vi "single_waveform_array_to_xy_array.vi"(1 "waveform in":waveform(dbl)) -> (0 "XY out":cluster{dbl[], "Y":dbl[]}(graph))   [LabVIEW 2020]
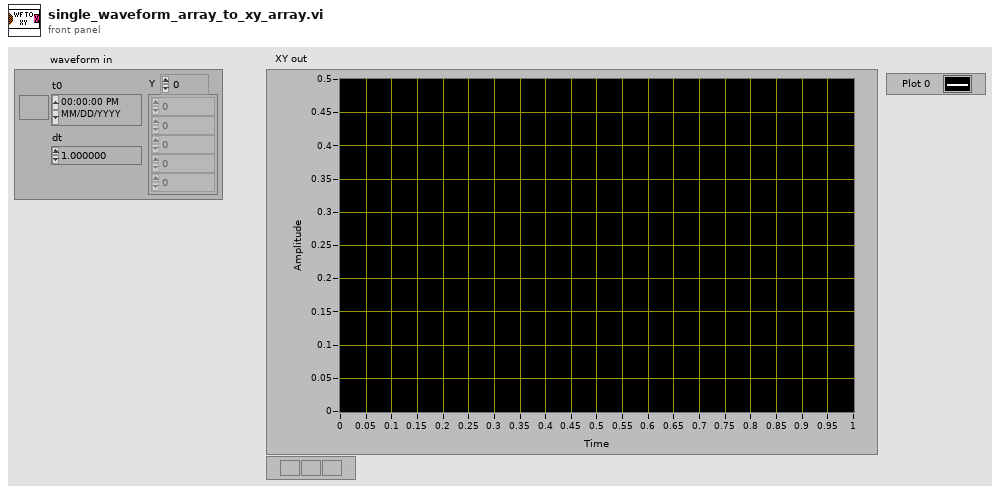
[diagram p1: front panel]
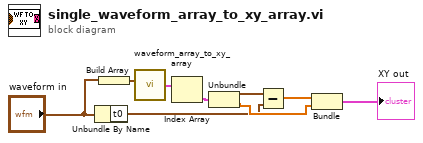
[diagram p0: block diagram]
diagram:
  n1 = Unbundle By Name("waveform in") -> ("t0"=w5:timestamp)
  n2 = Build Array("waveform in") -> (w1:waveform(dbl)[])
  n3 = call "waveform_array_to_xy_array.vi"("waveform array"=w1) -> ("XY array"=w2:cluster{timestamp[], "Y":dbl[]}[])  [unwired: 1 in]
  n4 = Index Array(array=w2) -> (element=w3:cluster{timestamp[], "Y":dbl[]})  [unwired: 1 in]
  n5 = Unbundle(w3) -> (w4:timestamp[], "Y"=w7:dbl[])
  n6 = Subtract(x=w4, y=w5) -> (x-y=w6:dbl[])
  n7 = Bundle(w6, "Y"=w7) -> (→"XY out":cluster{dbl[], "Y":dbl[]})  [unwired: 1 in]
